vi "Set Marker State.vi"(8 "Error In":errorcluster, 11 "Marker State In":T1) -> (0 "Error Out":errorcluster)   [LabVIEW 2014]
uses:
  Controls/GMap Marker State.ctl
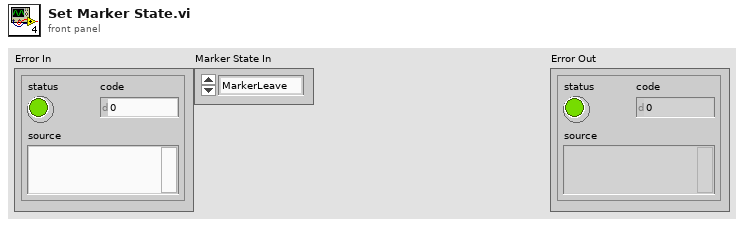
[diagram p1: front panel]
types:
  T1 = typedef "GMap Marker State.ctl" = enum16{"MarkerLeave", "MarkerEntered"}
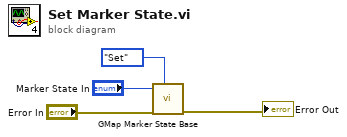
[diagram p0: block diagram]
diagram:
  n1 = call "GMap Marker State Base.vi"("Method"=enum16{"Get", "Set"}."Set", "Error In"="Error In", "Marker State In"="Marker State In") -> ("Error Out"=→"Error Out":errorcluster)  [unwired: 7 in, 1 out]
